vi "LXY.vi"() -> ()   [LabVIEW 2019]
uses:
  lib/Keithley 622x/Configure/2182 -A/Low Level/Typedefs/KE2182 -- Voltage Ranges.ctl
  lib/Keithley 622x/Configure/2182 -A/Low Level/Typedefs/KE2182 -- Filter Type.ctl
  lib/Keithley 622x/Configure/2182 -A/Low Level/Typedefs/KE2182 -- Filter Count.ctl
  lib/Keithley 622x/Configure/2182 -A/Low Level/Typedefs/KE2182 -- Filter Window.ctl
  lib/Keithley 622x/Configure/2182 -A/Low Level/Typedefs/KE2182 -- NPLCs.ctl
  lib/Keithley 622x/Configure/Delta PDelta DCon Modes/Typedefs/KE622x -- Delta Mode Params.ctl
  lib/Keithley 622x/Configure/Delta PDelta DCon Modes/Low Level/Typedefs/KE622x -- Delta PDelta Mode High Level.ctl
  lib/Keithley 622x/Configure/Delta PDelta DCon Modes/Low Level/Typedefs/KE622x -- Delta PDelta Mode Low Level.ctl
  lib/Keithley 622x/Configure/Delta PDelta DCon Modes/Low Level/Typedefs/KE622x -- Delta DCon Mode Delay.ctl
  lib/Keithley 622x/Configure/Delta PDelta DCon Modes/Low Level/Typedefs/KE622x -- Delta PDelta Mode Num Cycles Mode.ctl
  lib/Keithley 622x/Configure/Delta PDelta DCon Modes/Low Level/Typedefs/KE622x -- Delta PDelta Mode Num Cycles.ctl
  SubVI/initialize.lvlib
  SubVI.lvlib
  Take Seq.lvlib
  lib/Keithley 622x/Keithley 622x.lvlib
panel:
  in  "Delta Mode Params In":T1={"High Level (A)"=0.001, "Low Level (A)"=-0.001, "Delay (s)"=0.002, "Num Cycles Mode"=enum."Finite Count", "Finite Count"=10, "Abort On\nCompliance?"=FALSE, "Cold Swithing\nMode Enabled?"=FALSE} {"Finite Count" min=1 max=65536; "Low Level (A)" min=-0.105 max=0.0 format="%.3p"; "High Level (A)" min=0.0 max=0.105 format="%.3p"; "Delay (s)" min=0.001 max=9999.999 format="%.3f"}
  in  "2812 -A Params In":T12={"Auto Range?"=FALSE, "Man / Selected\nRange"=enum."10mV", "Enable Digital\nFilter?"=FALSE, "Filter Type"=enum."Moving", "Filter Count"=10, "Filter\nWindow (%)"=0.01, "Enable Analog\nFilter?"=FALSE, "NPLCs"=5} {"Filter\nWindow (%)" min=0.0 max=10.0 step=0.01 format="%.2f"; "Filter Count" min=1 max=100; "NPLCs" min=1 max=10}
  in  "Compliance  Level (A)":dbl=0.0001 format="%#_13g"
  in  "压电陶瓷电压 (0.1 Vpp)":dbl=0.1
  in  "6221 Resource":refnum<visa-resource-name>="GPIB0::10::INSTR"
  in  "2400 resource name":refnum<visa-resource-name>
  in  "33522b resource name":refnum<visa-resource-name>
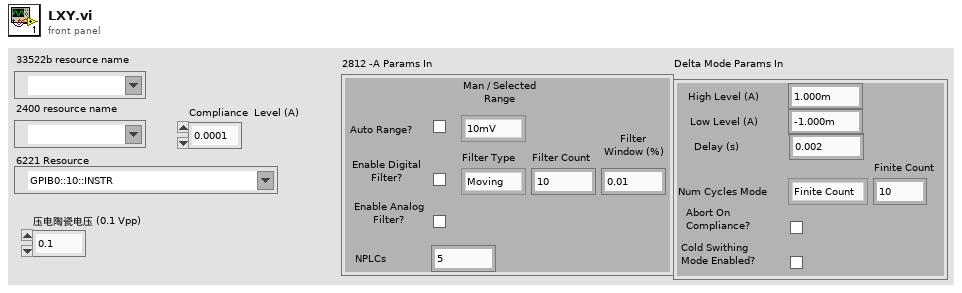
[diagram p1: front panel]
types:
  T1 = typedef "Keithley 622x.lvlib/KE622x -- Delta Mode Params.ctl" = cluster{"High Level (A)":T2, "Low Level (A)":T3, "Delay (s)":T4, "Num Cycles Mode":T5, "Finite Count":T6, "Abort On\nCompliance?":bool, "Cold Swithing\nMode Enabled?":bool}
  T2 = typedef "Keithley 622x.lvlib/KE622x -- Delta PDelta Mode High Level.ctl" = dbl
  T3 = typedef "Keithley 622x.lvlib/KE622x -- Delta PDelta Mode Low Level.ctl" = dbl
  T4 = typedef "Keithley 622x.lvlib/KE622x -- Delta DCon Mode Delay.ctl" = dbl
  T5 = typedef "Keithley 622x.lvlib/KE622x -- Delta PDelta Mode Num Cycles Mode.ctl" = enum16{"Finite Count", "Infinite"}
  T6 = typedef "Keithley 622x.lvlib/KE622x -- Delta PDelta Mode Num Cycles.ctl" = u32
  T7 = typedef "Keithley 622x.lvlib/KE2182 -- Voltage Ranges.ctl" = enum16{"10mV", "100mV", "1V", "10V", "100V"}
  T8 = typedef "Keithley 622x.lvlib/KE2182 -- Filter Type.ctl" = enum16{"Moving", "Repeat"}
  T9 = typedef "Keithley 622x.lvlib/KE2182 -- Filter Count.ctl" = u32
  T10 = typedef "Keithley 622x.lvlib/KE2182 -- Filter Window.ctl" = dbl
  T11 = typedef "Keithley 622x.lvlib/KE2182 -- NPLCs.ctl" = u32
  T12 = cluster{"Auto Range?":bool, "Man / Selected\nRange":T7, "Enable Digital\nFilter?":bool, "Filter Type":T8, "Filter Count":T9, "Filter\nWindow (%)":T10, "Enable Analog\nFilter?":bool, "NPLCs":T11}
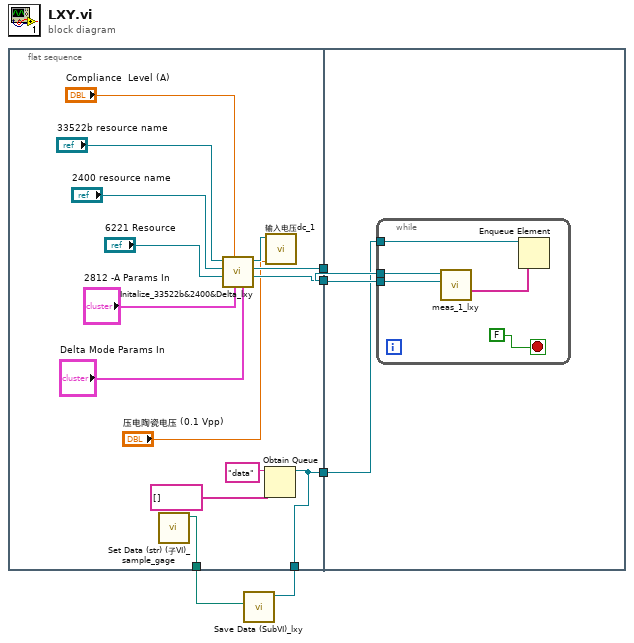
[diagram p0: block diagram]
diagram:
  n1 = flat-sequence {
    tunnel: [w15] -> w5
    tunnel: [w14] -> w4
    tunnel: [w7] -> w3
    tunnel: [w6] -> w2
    tunnel: [w7] -> w1
    tunnel: w3 -> [w20]
    tunnel: w4 -> [w21]
    tunnel: w5 -> [w22]
    frame #0 {
      n2 = call "Set Data (str) (子VI)_sample_gage.vi"() -> ("path"=w6:path)  [unwired: 10 in, 1 out]
      n3 = call "Initalize_33522b&2400&Delta_lxy.vi"("Delta Mode Params In"="Delta Mode Params In", "2812 -A Params In"="2812 -A Params In", "Compliance  Level (A)"="Compliance  Level (A)", "6221 Resource"="6221 Resource", "2400 resource name"="2400 resource name", "33522b resource name"="33522b resource name") -> ("6221 Resource 2"=w14:refnum<visa-resource-name>, "2400 resource name 2"=w15:refnum<visa-resource-name>, "33522b resource name 2"=w13:refnum<visa-resource-name>)  [unwired: 3 in]
      n4 = Obtain Queue(name (unnamed)="data", element data type=string[] [] ("数组")) -> (queue out=w7:refnum<queue>)  [unwired: 3 in, 2 out]
      n5 = call "输入电压dc_1.vi"("压电陶瓷电压 (0.1 Vpp)"="压电陶瓷电压 (0.1 Vpp)", "33522b resource name"=w13) -> ()  [unwired: 5 in]
    }
    frame #1 {
      n6 = while {
        tunnel: w22 -> [w27]
        tunnel: w21 -> [w26]
        tunnel: w20 -> [w24]
        stop <- FALSE stop-if-true
        n7 = call "meas_1_lxy.vi"("2400 resource name"=w27, "6221 Resource"=w26) -> ("数组"=w23:string[])  [unwired: 8 in, 1 out]
        n8 = Enqueue Element(queue=w24, element=w23) -> ()  [unwired: 2 in, 3 out]
      }
    }
  }
  n9 = call "Save Data (SubVI)_lxy.vi"("path"=w2, "队列输入"=w1) -> ()  [unwired: 10 in]
